vi "HandlerCounter.vi"(3 "error in":errorcluster, 4 "Reset Count":bool, 5 "Change in count":i16) -> (0 "error out":errorcluster, 2 "Count":i16)   [LabVIEW 2015]
doc: "Keeps count of anything you want. In this case it is meant to keep track of the number of registered event listeners so that we know when it's safe to destroy the event source (i.e., when this number = 0)\n\nSo you should call this with \"Reset Count\" = TRUE in the initialization code, and then with \"Change in count\" = +1 when registering new event listeners and = -1 when unregistering them. Then \"Count\" will return the current number of registered event listeners.\n\nNo error handling happens; the error in/error out is just to help you sequence your code using dataflow."
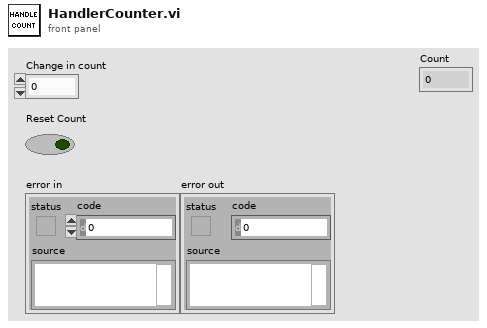
[diagram p1: front panel]
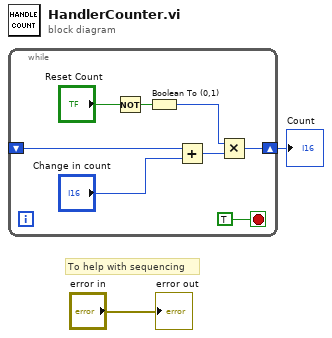
[diagram p0: block diagram]
diagram:
  # "To help with sequencing"
  n1 = while {
    shift-right: [w4] -> w2
    shift-left: _ -> [w3]
    stop <- TRUE ("stop") stop-if-true
    n2 = Not(x="Reset Count") -> (.not. x?=w9:bool)
    n3 = Boolean To (0,1)(Boolean=w9) -> (0, 1=w5:i16)
    n4 = Add(x=w3, y="Change in count") -> (x+y=w6:i16)
    n5 = Multiply(x=w5, y=w6) -> (x*y=w4:i16)
  }
  "Count" <- w2
  "error out" <- "error in"
